vi "singleAxisMultiMove_SingleAxis.vi"(0 "Bd ID":T4=1 min=1 max=32 step=1, 1 "Axis":T2=1 items=["Axis Control"=0, "Axis 1"=1, "Axis 2"=2, "Axis 3"=3, "Axis 4"=4, "Axis 5"=5, "Axis 6"=6, "Axis 7"=7, "Axis 8"=8, "Vector Space Control"=16, "Vector Space 1"=17, "Vector Space 2"=18, "Vector Space 3"=19, "Vector Space 4"=20, "Encoder Control"=32, "Encoder 1"=33, "Encoder 2"=34, "Encoder 3"=35, "Encoder 4"=36, "Encoder 5"=37, "Encoder 6"=38, "Encoder 7"=39, "Encoder 8"=40, "DAC Channel 1"=49, "DAC Channel 2"=50, "DAC Channel 3"=51, "DAC Channel 4"=52, "DAC Channel 5"=53, "DAC Channel 6"=54, "DAC Channel 7"=55, "DAC Channel 8"=56, "Stepper Output 1"=65, "Stepper Output 2"=66, "Stepper Output 3"=67, "Stepper Output 4"=68, "Stepper Output 5"=69, "Stepper Output 6"=70, "Stepper Output 7"=71, "Stepper Output 8"=72, "ADC Channel 1"=81, "ADC Channel 2"=82, "ADC Channel 3"=83, "ADC Channel 4"=84, "ADC Channel 5"=85, "ADC Channel 6"=86, "ADC Channel 7"=87, "ADC Channel 8"=88], 5 "error in (no error)":errorcluster, 7 "Target Positions":dbl[](array[numeric]), 8 "Stop Refnum":refnum<vi>, 9 "Trajectory Parameters":T1={"Operation Mode (Absolute)"=100, "Blend"=FALSE, "Velocity"=10.0, "Acceleration"=0.0, "Deceleration"=1000.0, "Blend Factor"=1, "Permitted Following Error"=0.0, "S Curve Time"=0} {"Operation Mode (Absolute)" items=["Absolute Position", "Relative Position"]; "Velocity" min=0.0 max=500.0 step=1.0}) -> (14 "Bd ID Out":T3, 15 "Resource Output":T2 items=["Axis Control"=0, "Axis 1"=1, "Axis 2"=2, "Axis 3"=3, "Axis 4"=4, "Axis 5"=5, "Axis 6"=6, "Axis 7"=7, "Axis 8"=8, "Vector Space Control"=16, "Vector Space 1"=17, "Vector Space 2"=18, "Vector Space 3"=19, "Vector Space 4"=20, "Encoder Control"=32, "Encoder 1"=33, "Encoder 2"=34, "Encoder 3"=35, "Encoder 4"=36, "Encoder 5"=37, "Encoder 6"=38, "Encoder 7"=39, "Encoder 8"=40, "DAC Channel 1"=49, "DAC Channel 2"=50, "DAC Channel 3"=51, "DAC Channel 4"=52, "DAC Channel 5"=53, "DAC Channel 6"=54, "DAC Channel 7"=55, "DAC Channel 8"=56, "Stepper Output 1"=65, "Stepper Output 2"=66, "Stepper Output 3"=67, "Stepper Output 4"=68, "Stepper Output 5"=69, "Stepper Output 6"=70, "Stepper Output 7"=71, "Stepper Output 8"=72, "ADC Channel 1"=81, "ADC Channel 2"=82, "ADC Channel 3"=83, "ADC Channel 4"=84, "ADC Channel 5"=85, "ADC Channel 6"=86, "ADC Channel 7"=87, "ADC Channel 8"=88], 19 "error out":errorcluster)   [LabVIEW 2010]
doc: "Iterates through the passed in array of target positions on the given axis using the given trajectory parameters. Function exits when one of the following occurs:\n\n-All moves have been completed\n-A kill stop is performed on the axis\n-A true condition is detected on the control pointed to by Stop Refnum\n-An error condition is detected\n\nNotes:\n\nAll operations are done on the host computer (no buffering or onboard programming).\n\nUses the FlexMotion \"Load Target Position.flx\" to send target positions to the controller board."
uses:
  <vilib>/Motion/FlexMotion/CustomControls/CustomControls.llb/Resource Out (Enum).flx
  Shared/typedefs/Trajectory Parameters.ctl
  <vilib>/Motion/FlexMotion/FunctionsVIs/Trajectory.llb/Load Accel/Decel in RPS/sec.flx
  <vilib>/Motion/FlexMotion/FunctionsVIs/StartStopMotion.llb/Blend Motion (8 axes).flx
  <vilib>/Motion/FlexMotion/FunctionsVIs/StartStopMotion.llb/Start Motion (8 axes).flx
  <vilib>/Motion/FlexMotion/FunctionsVIs/Trajectory.llb/Check Blend Complete Status (8 axes).flx
  <vilib>/Motion/FlexMotion/FunctionsVIs/Trajectory.llb/Check Move Complete Status (8 axes).flx
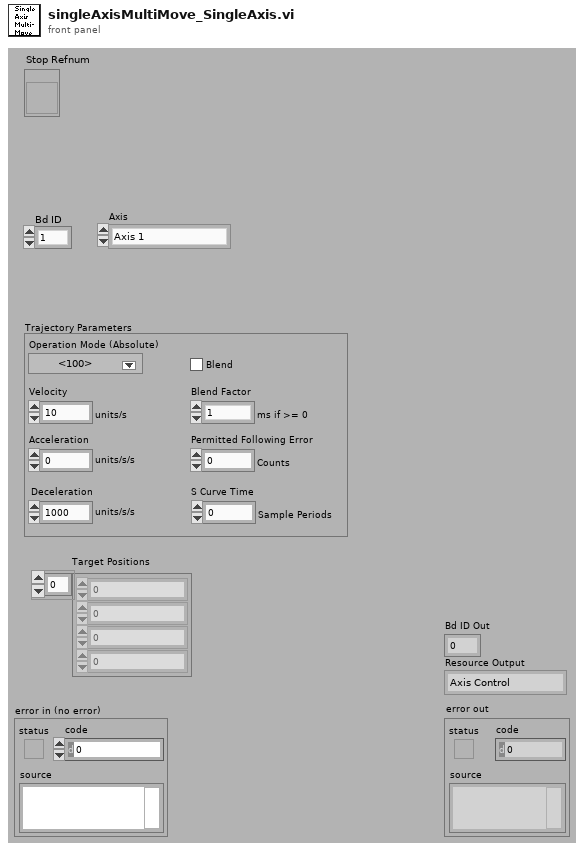
[diagram p1: front panel]
types:
  T1 = typedef "Trajectory Parameters.ctl" = cluster{"Operation Mode (Absolute)":u16, "Blend":bool, "Velocity":dbl, "Acceleration":dbl, "Deceleration":dbl, "Blend Factor":i16, "Permitted Following Error":dbl, "S Curve Time":u16}
  T2 = typedef "Resource Out (Enum).flx" = u16
  T3 = typedef "Bd Id Out" = u8
  T4 = typedef "Board Id" = u8
  T5 = cluster{"Run/Stop":bool, "Profile Complete":bool, "Motor Off ":bool, "Following Error":bool, "Limit Switch":bool, "Home Switch":bool, "SW Limit Switch":bool, "Watchdog":bool, "Velocity Threshold":bool, "Position Brkpt":bool, "Home Found":bool, "Index Found":bool, "High Speed Capture":bool, "Reverse Direction":bool, "Blend Complete":bool, "Move Complete":bool}
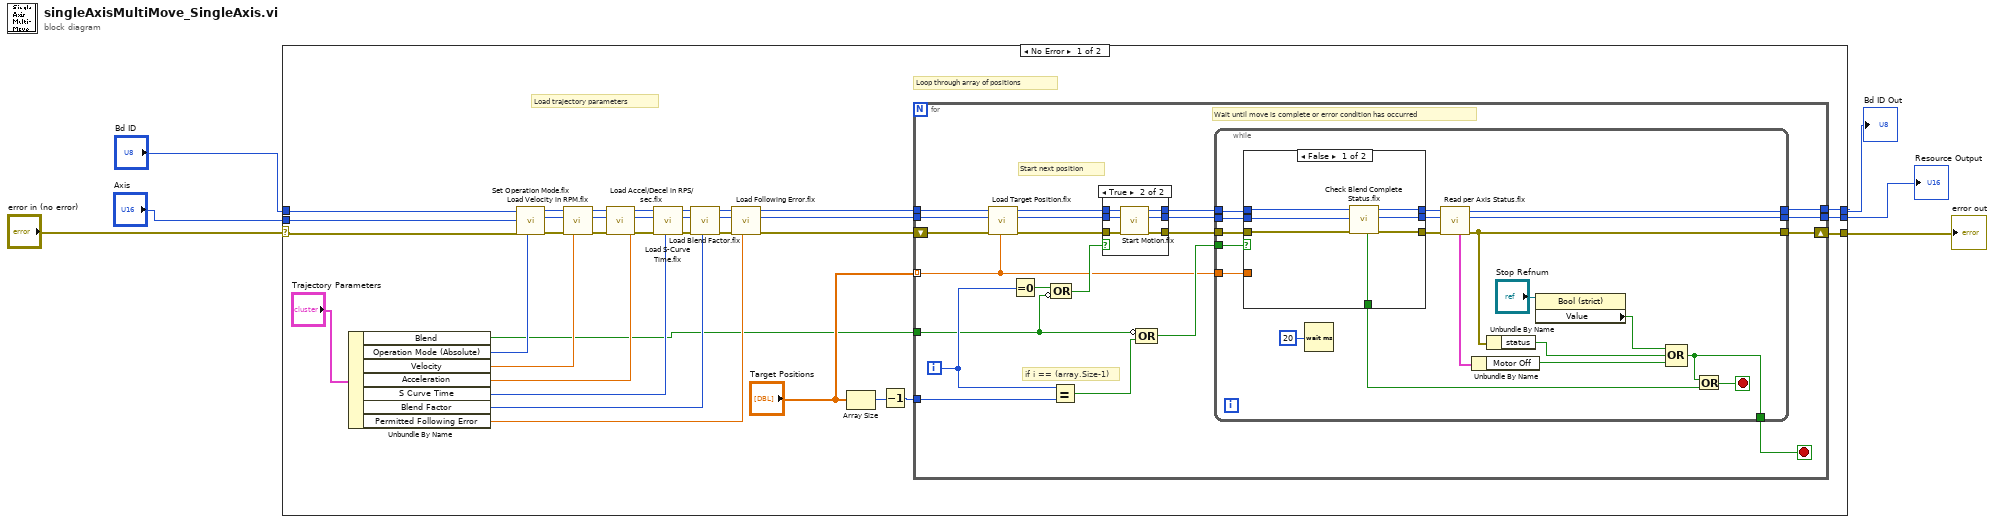
[diagram p0: block diagram]
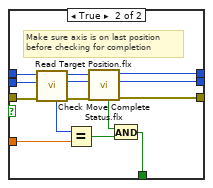
[diagram p2: hidden frame]
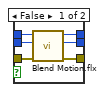
[diagram p3: hidden frame]
diagram:
  n1 = case shown="No Error" "error in (no error)" {
    selector: "error in (no error)" -> [w10 w116]
    tunnel: "Bd ID" -> [w41 w118]
    tunnel: "Axis" -> [w40 w117]
    tunnel: [w12 w116] -> w4
    tunnel: [w14 w117] -> w3
    tunnel: [w13 w118] -> w2
    frame No Error {
      # "Loop through array of positions"
      # "Load trajectory parameters"
      n2 = Unbundle By Name("Trajectory Parameters") -> ("Blend"=w7:bool, "Operation Mode (Absolute)"=w11:u16, "Velocity"=w21:dbl, "Acceleration"=w19:dbl, "S Curve Time"=w22:u16, "Blend Factor"=w15:i16, "Permitted Following Error"=w29:dbl)
      n3 = call <vilib>:"Set Operation Mode.flx"("Position Mode (Absolute)"=w11, "error in (no error)"=w10, "Axis or Vector Space"=w40, "Board ID"=w41) -> ("error out"=w37:errorcluster, "Resource Output"=w38:T2, "Bd ID Out"=w39:T3)  [unwired: 2 in]
      n4 = call <vilib>:"Load Velocity in RPM.flx"("Velocity (500)"=w21, "error in (no error)"=w37, "Axis or Vector Space"=w38, "Board ID"=w39) -> ("error out"=w18:errorcluster, "Resource Output"=w16:T2, "Bd ID Out"=w17:T3)  [unwired: 3 in]
      n5 = call "Load Accel/Decel in RPS/sec.flx"("Value (200)"=w19, "error in (no error)"=w18, "Axis or Vector Space"=w16, "Board ID"=w17) -> ("error out"=w23:errorcluster, "Resource Output"=w24:T2, "Bd ID Out"=w25:T3)  [unwired: 3 in]
      n6 = call <vilib>:"Load S-Curve Time.flx"("S Curve Time (1)"=w22, "error in (no error)"=w23, "Axis or Vector Space"=w24, "Board ID"=w25) -> ("error out"=w26:errorcluster, "Resource Output"=w27:T2, "Bd ID Out"=w28:T3)  [unwired: 3 in]
      n7 = call <vilib>:"Load Blend Factor.flx"("Blend Factor (-1)"=w15, "error in (no error)"=w26, "Axis or Vector Space"=w27, "Board ID"=w28) -> ("error out"=w36:errorcluster, "Resource Output"=w34:T2, "Bd ID Out"=w35:T3)  [unwired: 3 in]
      n8 = call <vilib>:"Load Following Error.flx"("Following Error"=w29, "error in (no error)"=w36, "Axis"=w34, "Board ID"=w35) -> ("error out"=w31:errorcluster, "Resource Output"=w32:T2, "Bd ID Out"=w33:T3)  [unwired: 3 in]
      n9 = Array Size(array="Target Positions") -> (size(s)=w9:i32)
      n10 = Decrement(x=w9) -> (x-1=w8:i32)
      n11 = for {
        shift-left: w31 -> [w57]
        shift-right: [w46] -> w12
        tunnel: "Target Positions" -> [w45] mode=indexing
        tunnel: w32 -> [w59]
        tunnel: w33 -> [w58]
        tunnel: [w47] -> w14
        tunnel: [w48] -> w13
        tunnel: w7 -> [w43]
        tunnel: w8 -> [w42]
        i -> [w51]
        stop <- w44 stop-if-true
        # "Start next position"
        # "if i == (array.Size-1)"
        # "Wait until move is complete or error condition has occurred"
        n12 = call <vilib>:"Load Target Position.flx"("Target Position (0)"=w45, "error in (no error)"=w57, "Axis"=w59, "Board ID"=w58) -> ("error out"=w60:errorcluster, "Resource Output"=w61:T2, "Bd ID Out"=w62:T3)  [unwired: 3 in]
        n13 = Equal To 0?(x=w51) -> (x = 0?=w50:bool)
        n14 = Compound Arithmetic op=OR(w50, invert w43) -> (w56:bool)
        n15 = Equal?(x=w51, y=w42) -> (x = y?=w55:bool)
        n16 = case shown="True" w56 {
          tunnel: w62 -> [w109 w115]
          tunnel: w61 -> [w108 w114]
          tunnel: w60 -> [w107 w113]
          tunnel: [w106 w112] -> w54
          tunnel: [w105 w111] -> w53
          tunnel: [w104 w110] -> w52
          frame False {
            n17 = call-poly <vilib>:"Blend Motion.flx"("error in (no error)"=w107, "Axis or Vector Space"=w108, "Board ID"=w109) -> ("error out"=w104:errorcluster, "Resource Output"=w105:T2, "Bd ID Out"=w106:T3)  [unwired: 3 in]
          }
          frame True {
            n18 = call-poly <vilib>:"Start Motion.flx"("error in (no error)"=w113, "Axis or Vector Space"=w114, "Board ID"=w115) -> ("error out"=w110:errorcluster, "Resource Output"=w111:T2, "Bd ID Out"=w112:T3)  [unwired: 3 in]
          }
        }
        n19 = Compound Arithmetic op=OR(invert w43, w55) -> (w49:bool)
        n20 = while {
          tunnel: w54 -> [w69]
          tunnel: w53 -> [w68]
          tunnel: w52 -> [w67]
          tunnel: [w74] -> w46
          tunnel: [w77] -> w47
          tunnel: [w78] -> w48
          tunnel: [w70] -> w44
          tunnel: w49 -> [w66]
          tunnel: w45 -> [w65]
          stop <- w81 stop-if-true
          n21 = case shown="False" w66 {
            tunnel: w67 -> [w87 w98]
            tunnel: w68 -> [w88 w99]
            tunnel: w69 -> [w89 w100]
            tunnel: [w86 w101] -> w79
            tunnel: [w84 w103] -> w76
            tunnel: [w85 w102] -> w75
            tunnel: [w83 w94] -> w71
            tunnel: w65 -> [_ w92]
            frame False {
              n22 = call-poly <vilib>:"Check Blend Complete Status.flx"("error in (no error)"=w87, "Axis or Vector Space"=w88, "Board ID"=w89) -> ("error out"=w86:errorcluster, "Resource Output"=w85:T2, "Bd ID Out"=w84:T3, "Blend Complete"=w83:bool)  [unwired: 3 in]
            }
            frame True {
              # "Make sure axis is on last position\nbefore checking for completion"
              n23 = call <vilib>:"Read Target Position.flx"("error in (no error)"=w98, "Axis"=w99, "Board ID"=w100) -> ("error out"=w97:errorcluster, "Resource Output"=w96:T2, "Bd ID Out"=w95:T3, "Target Position"=w93:i32)  [unwired: 3 in]
              n24 = Equal?(x=w93, y=w92) -> (x = y?=w91:bool)
              n25 = call-poly <vilib>:"Check Move Complete Status.flx"("error in (no error)"=w97, "Axis or Vector Space"=w96, "Board ID"=w95) -> ("error out"=w101:errorcluster, "Resource Output"=w102:T2, "Bd ID Out"=w103:T3, "Move Complete"=w90:bool)  [unwired: 3 in]
              n26 = And(x=w90, y=w91) -> (x .and. y?=w94:bool)
            }
          }
          n27 = Wait (ms)(milliseconds to wait=u32 20) -> ()  [unwired: 1 out]
          n28 = call <vilib>:"Read per Axis Status.flx"("error in (no error)"=w79, "Axis"=w75, "Board ID"=w76) -> ("error out"=w74:errorcluster, "Resource Output"=w77:T2, "Bd ID Out"=w78:T3, "Per Axis H/W Status"=w82:T5)  [unwired: 3 in]
          n29 = Unbundle By Name(w82) -> ("Motor Off"=w73:bool)
          n30 = Unbundle By Name(w74) -> ("status"=w72:bool)
          n31 = property class="Bool (strict)"(reference="Stop Refnum") -> ("Value"=w63:bool)  [unwired: 1 in, 2 out]
          n32 = Compound Arithmetic op=OR(w63, w72, w73) -> (w70:bool)
          n33 = Or(x=w70, y=w71) -> (x .or. y?=w81:bool)
        }
      }
    }
    frame Error {
    }
  }
  "error out" <- w4
  "Bd ID Out" <- w2
  "Resource Output" <- w3
